vi "Convert Unit (DBL).vi"(4 "Quantity":T1, 5 "error in (no error)":errorcluster, 6 "Target Unit":T2, 7 "Base Unit":T2, 8 "Data":dbl) -> (0 "error out":errorcluster, 3 "Converted Data":dbl)   [LabVIEW 2023, in "NI_HFNetworkAnalysis.lvlib"]
doc: "Convert data for a specified quantity from a base unit to a new unit."
uses:
  NI_HFNetworkAnalysis.lvlib
  Controls/Unit.ctl
  Controls/Quantity.ctl
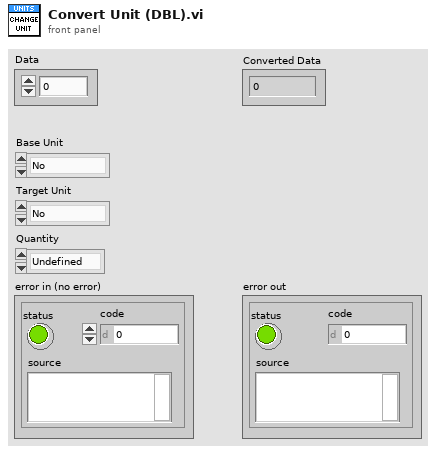
[diagram p1: front panel]
types:
  T1 = typedef "NI_HFNetworkAnalysis.lvlib/Quantity.ctl" = enum16{"Undefined", "V", "I", "A", "B", "P", "Z", "PowerRatio", "Gamma", "Index"}
  T2 = typedef "NI_HFNetworkAnalysis.lvlib/Unit.ctl" = enum16{"No", "s", "Hz", "V", "A", "Ohm", "W", "dB", "dBV", "dBA", "dBm", "percent", "rad", "deg"}
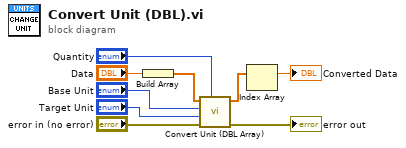
[diagram p0: block diagram]
diagram:
  n1 = Build Array("Data") -> (w2:dbl[])
  n2 = call "Convert Unit (DBL Array).vi"("Quantity"="Quantity", "error in (no error)"="error in (no error)", "Target Unit"="Target Unit", "Base Unit"="Base Unit", "Data"=w2) -> ("error out"=→"error out":errorcluster, "Converted Data"=w3:dbl[])  [unwired: 2 in]
  n3 = Index Array(array=w3) -> (element=→"Converted Data":dbl)  [unwired: 1 in]
